vi "API Demo.vi"() -> ()   [LabVIEW 2024]
uses:
  <vilib>/addons/_JKI.lib/REST Client/classes/REST Client/HTTP Header.ctl
  <vilib>/NI/Advanced HTTP Client/Header--Combo Box.ctl
  <vilib>/addons/_JKI.lib/REST Client/classes/REST Client/REST Client.lvclass
  <vilib>/NI/Advanced HTTP Client/Session.lvclass
panel:
  out "Response body 2":string
  in  "Path 2":string
  out "Parsed JSON":T1
  out "Response body":string
  out "Status String":string
  out "error out":errorcluster
  in  "Path":string="/api/search/components?search_string=ID%3E4%2Chas_test%3DSensor%20IV%20-%20Vendor"
  in  "Default Headers ([JSON])":T2[](array[typedef])=[{"header"="Content-Type", "value"="application/json"}, {"header"="Authorization", "value"="Bearer eyJhbGciOiJIUzI1NiIsInR5cCI6IkpXVCJ9.eyJ1c2VyX2lkIjoyLCJleHAiOjE3MzkwNTM2NzV9.igKE6g_W7AM7HyktJz4-b3a72s0kWm6g0pQc-QG5k84"}]
  in  "Base URL":string="https://prod-etl.app.cern.ch"
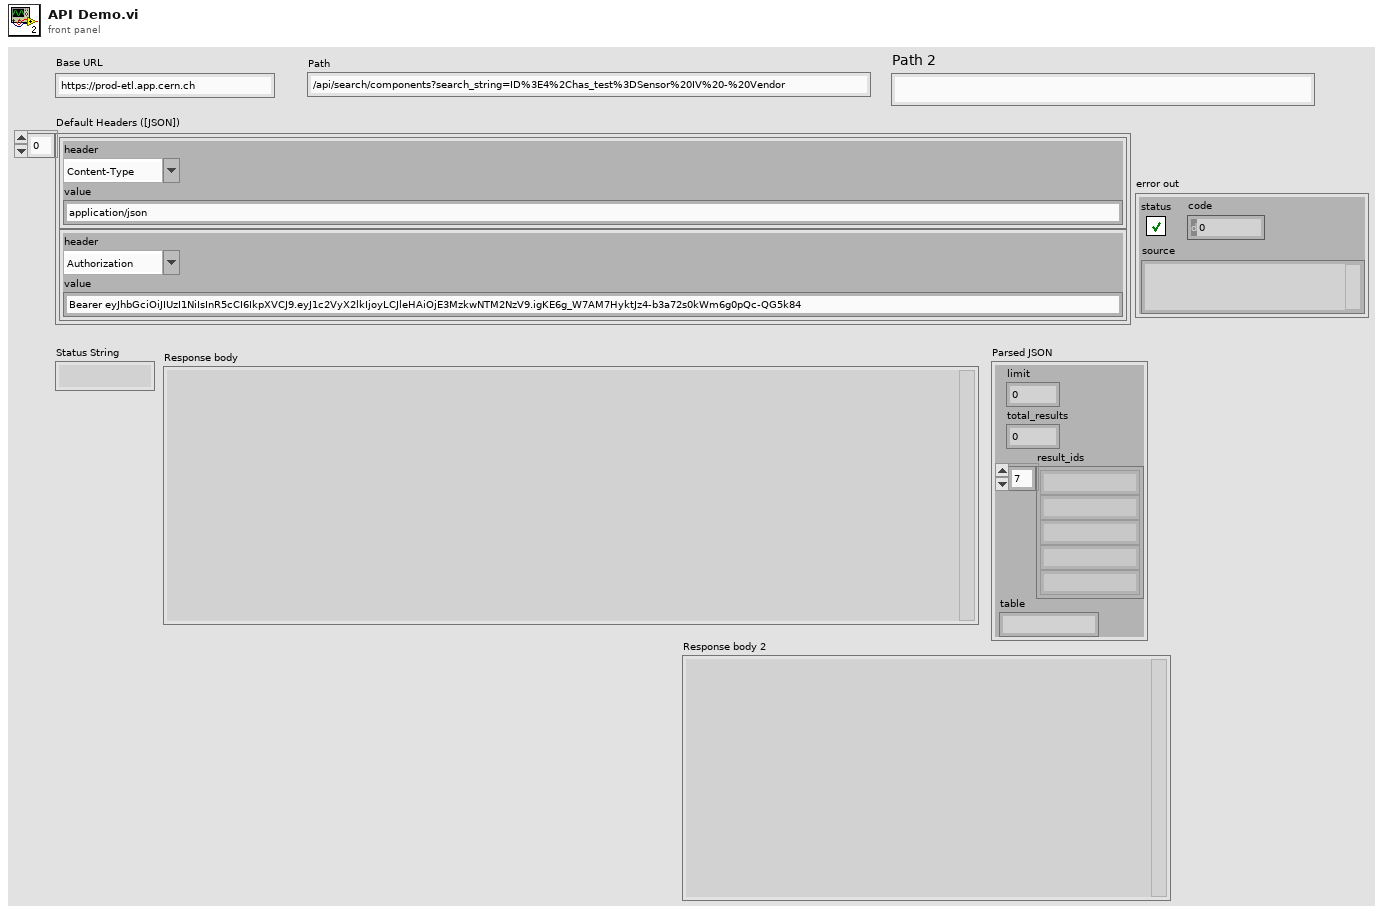
[diagram p1: front panel]
types:
  T1 = cluster{"limit":i32, "total_results":i32, "result_ids":string[], "table":string}
  T2 = typedef "REST Client.lvlib/REST Client.lvclass/HTTP Header.ctl" = cluster{"header":T3, "value":string}
  T3 = typedef "lib_NI_Advanced HTTP Client.lvlib/Session.lvclass/Header--Combo Box.ctl" = string
  T4 = cluster{"limit":i32, "total_results":i32, "results_ids":string[], "table":string}
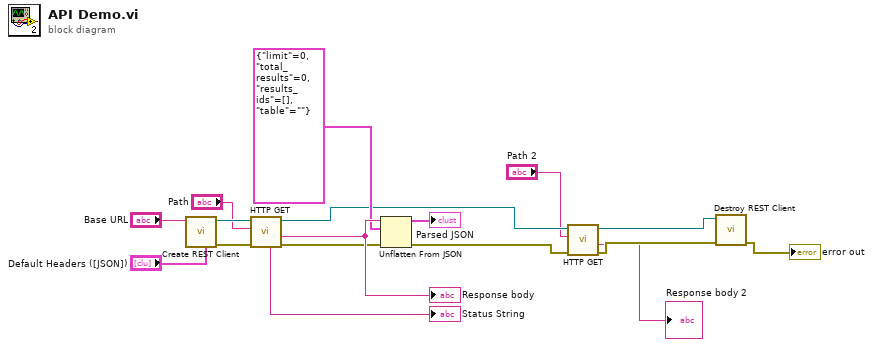
[diagram p0: block diagram]
diagram:
  n1 = call <vilib>:"Create REST Client.vi"("Default Headers ([JSON])"="Default Headers ([JSON])", "Base URL"="Base URL") -> ("error out"=w14:errorcluster, "REST Client out"=w15:refnum<class "REST Client.lvclass">)  [unwired: 8 in]
  n2 = call-dynamic "HTTP GET.vi"("error in (no error)"=w14, "Path"="Path", "REST Client in"=w15) -> ("error out"=w8:errorcluster, "Response body"=w11:string, "REST Client out"=w7:refnum<class "REST Client.lvclass">, "Status String"=→"Status String":string)  [unwired: 3 in, 2 out]
  "Response body" <- w11
  n3 = Unflatten From JSON(JSON string=w11, type and defaults=T4 {"limit"=0, "total_results"=0, "results_ids"=[], "table"=""}, error in (no error)=w8) -> (value=→"Parsed JSON":T4, error out=w5:errorcluster)  [unwired: 4 in]
  n4 = call-dynamic "HTTP GET.vi"("error in (no error)"=w5, "Path"="Path 2", "REST Client in"=w7) -> ("error out"=w4:errorcluster, "Response body"=→"Response body 2":string, "REST Client out"=w6:refnum<class "REST Client.lvclass">)  [unwired: 3 in, 3 out]
  n5 = call-dynamic "Destroy REST Client.vi"("error in (no error)"=w4, "REST Client in"=w6) -> ("error out"=→"error out":errorcluster)  [unwired: 9 in]
